vi "Get topic.vi"(11 "ISubscribe in":refnum<class "ISubscribe.lvclass">) -> (2 "Topic":string, 3 "ISubscribe out":refnum<class "ISubscribe.lvclass">)   [LabVIEW 2020, in "wamplv.lvlib" / "ISubscribe.lvclass"]
uses:
  ISubscribe.lvclass
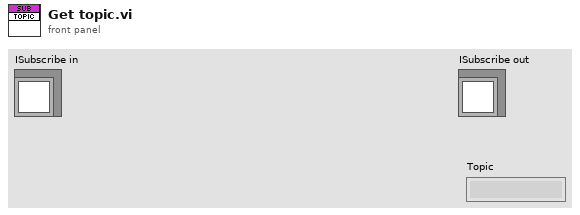
[diagram p1: front panel]
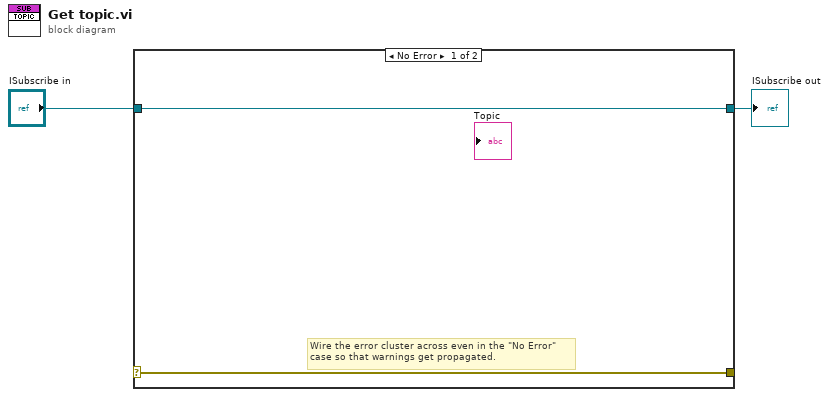
[diagram p0: block diagram]
diagram:
  n1 = case shown="No Error" w4 {
    selector: [w5 w8] -> w4
    tunnel: [w5 w8] -> w3
    tunnel: [w6 w7] -> w1
    tunnel: "ISubscribe in" -> [w6 w7]
    frame No Error {
      # "Wire the error cluster across even in the \"No Error\"\ncase so that warnings get propagated."
    }
    frame Error {
    }
  }
  "ISubscribe out" <- w1
